vi "SetTextureBlendMode.vi"(8 "No Error":errorcluster, 10 "Blend Mode":T1 items=["SDL_BLENDMODE_NONE"=0, "SDL_BLENDMODE_BLEND"=1, "SDL_BLENDMODE_BLEND_PREMULTIPLIED"=16, "SDL_BLENDMODE_ADD"=2, "SDL_BLENDMODE_ADD_PREMULTIPLIED"=32, "SDL_BLENDMODE_MOD"=4, "SDL_BLENDMODE_MUL"=8, "SDL_BLENDMODE_INVALID"=2147483647], 11 "Texture [SDL_Texture *]":i64 format="%.0x") -> (0 "error out":errorcluster)   [LabVIEW 2024, in "SDL3.lvlib" / "Render.lvlib"]
doc: "<B>Summary</B>\nSet the blend mode for a texture, used by <B>SDL_RenderTexture()</B>.\n\n<B>Remarks</B>\nIf the blend mode is not supported, the closest supported mode is chosen and this function returns false."
uses:
  Render.lvlib
  Blendmode/BlendMode--ring.ctl
  <vilib>/Utility/error.llb/Error Cluster From Error Code.vi
  Error/Error.lvlib
  Lib/Win32/SDL3.dll
  Blendmode/Blendmode.lvlib
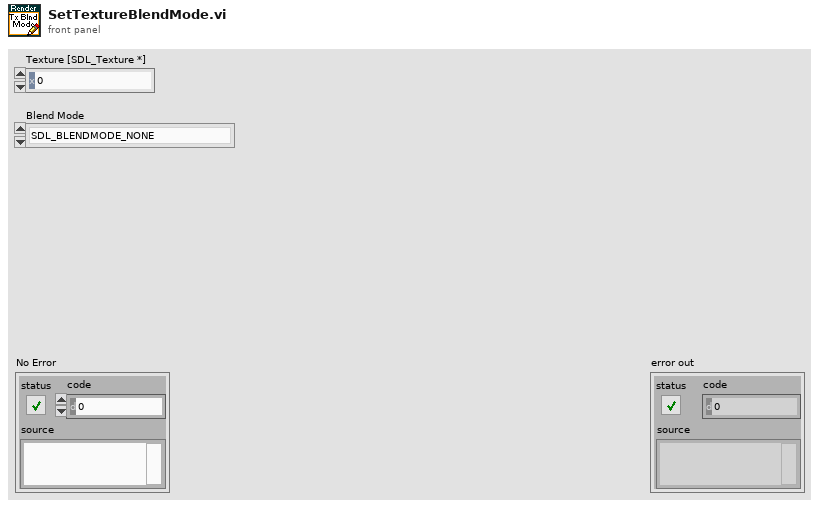
[diagram p1: front panel]
types:
  T1 = typedef "SDL3.lvlib/Blendmode.lvlib/BlendMode--ring.ctl" = u32
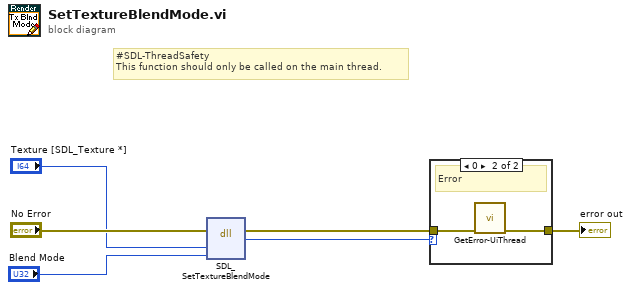
[diagram p0: block diagram]
diagram:
  # "#SDL-ThreadSafety\nThis function should only be called on the main thread."
  n1 = dll-call lib="C:/Users/Thomas/Documents/Projects/LV-SDL3/Lib/Win32/SDL3.dll" fn="SDL_SetTextureBlendMode"(error in="No Error", "texture"="Texture [SDL_Texture *]", "blendmode"="Blend Mode") -> (error out=w5:errorcluster, "return type"=w3:i32)  [unwired: 4 in, 1 out]
  n2 = case shown="0" w3 {
    tunnel: w5 -> [w7 w9]
    tunnel: [w7 w8] -> w4
    frame Default {
      # "Ok"
    }
    frame 0 {
      # "Error"
      n3 = call "GetError-UiThread.vi"("No Error"=w9) -> ("error out"=w8:errorcluster)  [unwired: 10 in]
    }
  }
  "error out" <- w4
